vi "Write_Html_Report_webserver.vi"(0 "Report inputs":T1={"Remarks"="", "Verdict"="", "Status Code"=0, "Status Description"="", "JazzDashboardLink"="", "ReprtPath"="", "Timestamp"="", "TestSuite"="", "TestCase"="", "Iterations"=0, "Time taken to execute  test in msec"="", "Delay Between Iterations"=1000}, 5 "Error In":errorcluster) -> (19 "Error Out":errorcluster)   [LabVIEW 2017]
doc: "HTML Report:\n1. This SubVI accepts string inputs and creates the HTML report\n 2. Store it in location below \n C:\\Integration_Workspace\\Test_Component\\Ultrasonic_Test_Scripts\\Result_Next_Gen\\ReportTC_TestcasenameDate_DDMMYY_Time_HH_MM_SS.html\n3. After test case execution, HTML report will be uploaded to RQM, and linked to execution record id of the test case."
uses:
  html_report_cluster.ctl
  <vilib>/Utility/NIReport.llb/HTML Report Text Alignment.ctl
  <vilib>/Utility/NIReport.llb/Append Report Text (str wrap).vi
  <vilib>/Utility/NIReport.llb/Append Text Table to Report (wrap).vi
  <vilib>/printing/ReportDocExtensions.llb/Append Front Panel Image to Report (string).vi
  <vilib>/Utility/NIReport.llb/NI_report.lvclass
  <vilib>/Utility/NIReport.llb/NI_ReportGenerationCore.lvlib
panel:
  # "INPUT"
  # "ERROR"
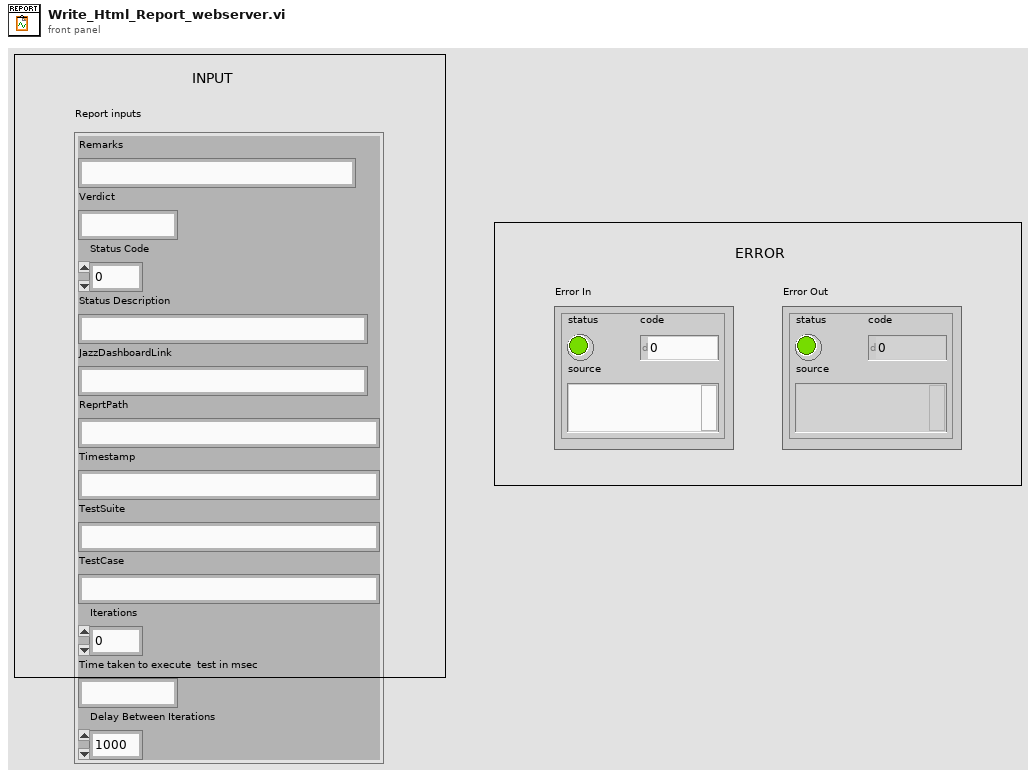
[diagram p1: front panel]
types:
  T1 = typedef "html_report_cluster.ctl" = cluster{"Remarks":string, "Verdict":string, "Status Code":i32, "Status Description":string, "JazzDashboardLink":string, "ReprtPath":string, "Timestamp":string, "TestSuite":string, "TestCase":string, "Iterations":i64, "Time taken to execute  test in msec":string, "Delay Between Iterations":i64}
  T2 = typedef "NI_ReportGenerationCore.lvlib/HTML Report Text Alignment.ctl" = enum16{"(default)", "LEFT", "CENTER", "RIGHT"}
  T3 = enum16{"Standard Report", "HTML", "Word", "Excel"}
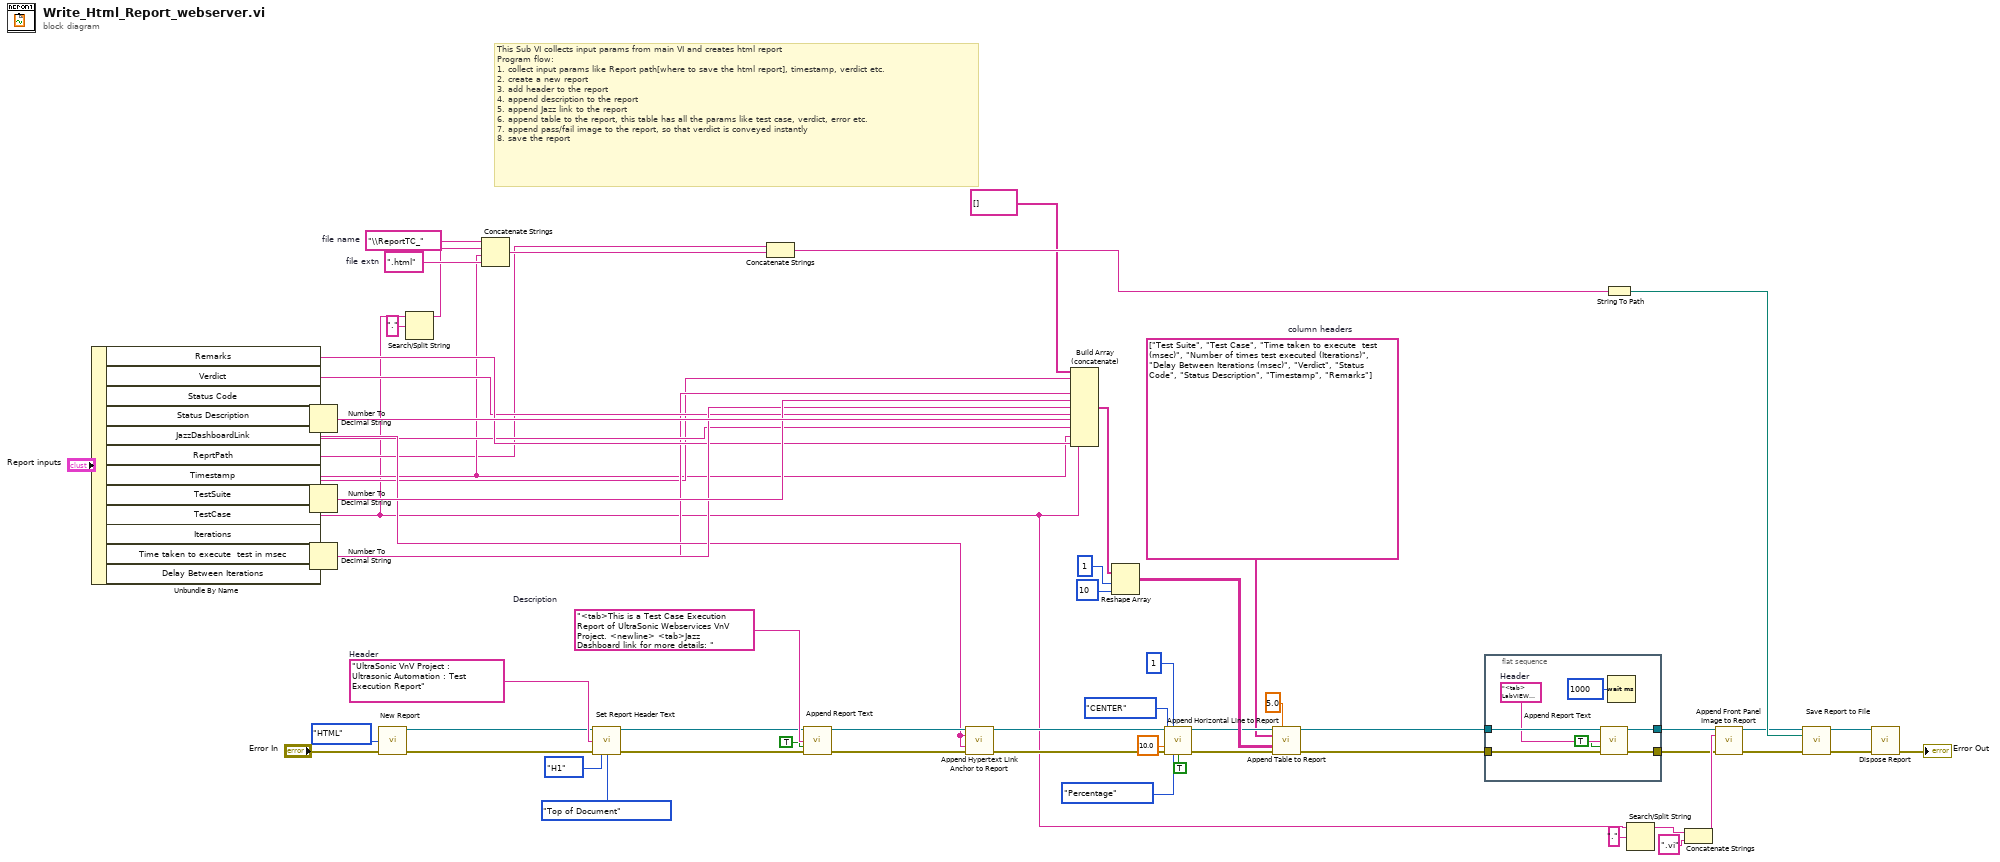
[diagram p0: block diagram]
diagram:
  w8 = "\\ReportTC_"  # file name
  w44 = "<tab>This is a Test Case Execution Report of UltraSonic Webservices VnV Project. <newline> <tab>Jazz Dashboard link for more details: "  # Description
  w40 = "UltraSonic VnV Project : Ultrasonic Automation : Test Execution Report"  # Header
  w63 = ".html"  # file extn
  w49 = string[] ["Test Suite", "Test Case", "Time taken to execute  test (msec)", "Number of times test executed (Iterations)", "Delay Between Iterations (msec)", "Verdict", "Status Code", "Status Description", "Timestamp", "Remarks"]  # column headers
  # "This Sub VI collects input params from main VI and creates html report\nProgram flow:\n1. collect input params like Report path[where to save the html report], timestamp, verdict etc.\n2. create a new report \n3. add header to the report\n4. append description to the report\n5. append Jazz link to the report\n6. append table to the report, this table has all the params like test case, verdict, error etc.\n7. append pass/fail image to the report, so that verdict is conveyed instantly\n8. save the report"
  n1 = Unbundle By Name("Report inputs") -> ("Remarks"=w33:string, "Verdict"=w30:string, "Status Code"=w31:i32, "Status Description"=w32:string, "JazzDashboardLink"=w34:string, "ReprtPath"=w24:string, "Timestamp"=w25:string, "TestSuite"=w26:string, "TestCase"=w7:string, "Iterations"=w28:i64, "Time taken to execute  test in msec"=w27:string, "Delay Between Iterations"=w29:i64)
  n2 = Number To Decimal String(number=w31) -> (decimal integer string=w65:string)  [unwired: 1 in]
  n3 = Number To Decimal String(number=w28) -> (decimal integer string=w37:string)  [unwired: 1 in]
  n4 = Number To Decimal String(number=w29) -> (decimal integer string=w36:string)  [unwired: 1 in]
  n5 = call <vilib>:"New Report.vi"("report type"=T3."HTML", "error in (no error)"="Error In") -> ("report out"=w39:refnum<class "NI_report.lvclass">, "error out"=w38:errorcluster)  [unwired: 12 in]
  n6 = Search/Split String(string=w7, search string/char (-)=".") -> (substring before match=w5:string)  [unwired: 1 in, 2 out]
  n7 = Concatenate Strings "Concatenate Strings"(w8, w5, w25, w63) -> (w62:string)
  n8 = call-dynamic "Set Report Header Text.vi"("report in"=w39, "center header text"=w40, "error in (no error)"=w38, "HTML header size"=enum16{"H1", "H2", "H3", "H4", "H5", "H6", "H7"}."H1", "header placement"=enum16{"Top of Document", "Append to Body"}."Top of Document") -> ("report out"=w43:refnum<class "NI_report.lvclass">, "error out"=w46:errorcluster)  [unwired: 9 in]
  n9 = Concatenate Strings "Concatenate Strings"(w24, w62) -> (w64:string)
  n10 = call-poly <vilib>:"Append Report Text.vi"("report in"=w43, "text"=w44, "append on new line? (F)"=TRUE, "error in (no error)"=w46) -> ("report out"=w50:refnum<class "NI_report.lvclass">, "error out"=w51:errorcluster)  [unwired: 8 in, 2 out]
  n11 = call-dynamic "Append Hypertext Link Anchor to Report.vi"("report in"=w50, "URL of link - href"=w34, "link text"=w34, "error in (no error)"=w51) -> ("report out"=w55:refnum<class "NI_report.lvclass">, "error out"=w54:errorcluster)  [unwired: 8 in, 2 out]
  n12 = Build Array (concatenate)(string[] [] ("array"), w26, w7, w27, w37, w36, w30, w65, w32, w25, w33) -> (w57:string[])
  n13 = Reshape Array "Reshape Array"(w57, 1 ("dimension size"), 10 ("dimension size")) -> (w60:string[][])
  n14 = call-dynamic "Append Horizontal Line to Report.vi"("report in"=w55, "size (default)"=1, "align (default)"=HTML_Report_Text_Alignment."CENTER", "width (100=default)"=10.0, "error in (no error)"=w54, "width units"=enum16{"Pixels", "Percentage"}."Percentage", "noshade (F)"=TRUE) -> ("report out"=w52:refnum<class "NI_report.lvclass">, "error out"=w53:errorcluster)  [unwired: 7 in]
  n15 = call-poly <vilib>:"Append Table to Report.vi"("report in"=w52, "column width (1)"=5.0, "column headers"=w49, "text data"=w60, "error in (no error)"=w53) -> ("report out"=w2:refnum<class "NI_report.lvclass">, "error out"=w1:errorcluster)  [unwired: 7 in, 2 out]
  n16 = flat-sequence {
    tunnel: [w72] -> w4
    tunnel: [w71] -> w3
    tunnel: w2 -> [w70]
    tunnel: w1 -> [w69]
    frame #0 {
      w68 = "<tab> LabVIEW FRONT PANEL RESULT<newline>"  # Header
      n17 = call-poly <vilib>:"Append Report Text.vi"("report in"=w70, "text"=w68, "append on new line? (F)"=TRUE, "error in (no error)"=w69) -> ("report out"=w72:refnum<class "NI_report.lvclass">, "error out"=w71:errorcluster)  [unwired: 8 in, 2 out]
      n18 = Wait (ms)(milliseconds to wait=u32 1000) -> ()  [unwired: 1 out]
    }
  }
  n19 = String To Path(string=w64) -> (path=w61:path)
  n20 = Search/Split String(string=w7, search string/char (-)=".") -> (substring before match=w19:string)  [unwired: 1 in, 2 out]
  n21 = Concatenate Strings(w19, ".vi" ("string")) -> (w17:string)
  n22 = call-poly <vilib>:"Append Front Panel Image to Report.vi"("report in"=w4, "VI"=w17, "error in (no error)"=w3) -> ("report out"=w21:refnum<class "NI_report.lvclass">, "error out"=w16:errorcluster)  [unwired: 8 in, 3 out]
  n23 = call-dynamic "Save Report to File.vi"("report in"=w21, "report file path"=w61, "error in (no error)"=w16) -> ("report out"=w48:refnum<class "NI_report.lvclass">, "error out"=w47:errorcluster)  [unwired: 11 in]
  n24 = call-dynamic "Dispose Report.vi"("report in"=w48, "error in (no error)"=w47) -> ("error out"=→"Error Out":errorcluster)  [unwired: 13 in]
